vi "Ver 3.0.vi"() -> ()   [LabVIEW 2016]
doc: "This example VI shows how to use thermocouples to take a temperature measurement.\n\nNote:\nFor front panel measurements, make sure the Input switch is in the out position(F)\nFor plug-in card measurements, make sure the Input switch is in the in poisition(R)"
uses:
  Documents/keithley_27xx/Keithley 27XX/Public/Configure/Measurement Specific/Configure FRTD.vi
  Documents/keithley_27xx/Keithley 27XX/Public/Configure/Measurement Specific/Configure Thermocouple.vi
  Documents/keithley_27xx/Keithley 27XX/Public/Configure/Measurement Specific/Configure Thermistor.vi
  Documents/keithley_27xx/Keithley 27XX/Public/Data/Read Multiple Direct.vi
  Documents/keithley_27xx/Keithley 27XX/Keithley 27XX.lvlib
  Documents/keithley_27xx/Keithley 27XX/Public/Close.vi
panel:
  out "Timestamp 12":dbl[](array[numeric])
  out "Timestamp 11":dbl[](array[numeric])
  out "Timestamp 10":dbl[](array[numeric])
  out "Timestamp 9":dbl[](array[numeric])
  out "Timestamp 8":dbl[](array[numeric])
  out "Timestamp 7":dbl[](array[numeric])
  out "Timestamp 6":dbl[](array[numeric])
  out "Timestamp 5":dbl[](array[numeric])
  out "Timestamp 4":dbl[](array[numeric])
  out "Timestamp 3":dbl[](array[numeric])
  out "Timestamp 2":dbl[](array[numeric])
  out "Measurement 12":dbl[](array[numeric])
  out "Measurement 11":dbl[](array[numeric])
  out "Measurement 10":dbl[](array[numeric])
  out "Measurement 9":dbl[](array[numeric])
  out "Measurement 8":dbl[](array[numeric])
  out "Measurement 7":dbl[](array[numeric])
  out "Measurement 6":dbl[](array[numeric])
  out "Measurement 5":dbl[](array[numeric])
  out "Measurement 4":dbl[](array[numeric])
  out "Measurement 3":dbl[](array[numeric])
  out "Measurement 2":dbl[](array[numeric])
  out "Timestamp 1":dbl[](array[numeric])
  out "Measurement 1":dbl[](array[numeric])
  in  "# of Channels":dbl=3.0
  in  "Sample size":dbl=3.0
  in  "Sensor Type":string(combo)="Thermistor"
  in  "Delta1":dbl=1.0
  in  "Beta1":dbl=0.1
  in  "Alpha1":dbl=0.0038
  in  "Serial Configuration":T1={"Baud Rate (9600)"=9600, "Flow Control (1: XON/XOFF)"=1, "Termination Char (0:CR)"=0} {"Termination Char (0:CR)" items=["CR", "LF", "CRLF (Do not use)", "LFCR (Do not use)"]; "Flow Control (1: XON/XOFF)" items=["None", "XON/XOFF", "RTS/CTS (2701 Only)", "XON/XOFF & RTS/CTS (2701 Only)"]; "Baud Rate (9600)" items=["300"=300, "600"=600, "1200"=1200, "2400"=2400, "4800"=4800, "9600"=9600, "19.2k"=19200, "38.4k (2701 Only)"=38400, "57.6k (2701 Only)"=57600, "115.2k (2701 Only)"=115200]}
  in  "VISA resource name":refnum<visa-resource-name>="TCPIP0::192.168.69.200::1394::SOCKET"
  in  "Channels":string="101,102,103"
  in  "Temperature (0: Celsius)":u16(ring) items=["Celsius", "Fahrenheit", "Kelvin"]
  # "*For front panel measurements, make sure the Input switch is in the out position(F)*\n  For plug-in card measurements, make sure the Input switch is in the in position(R)"
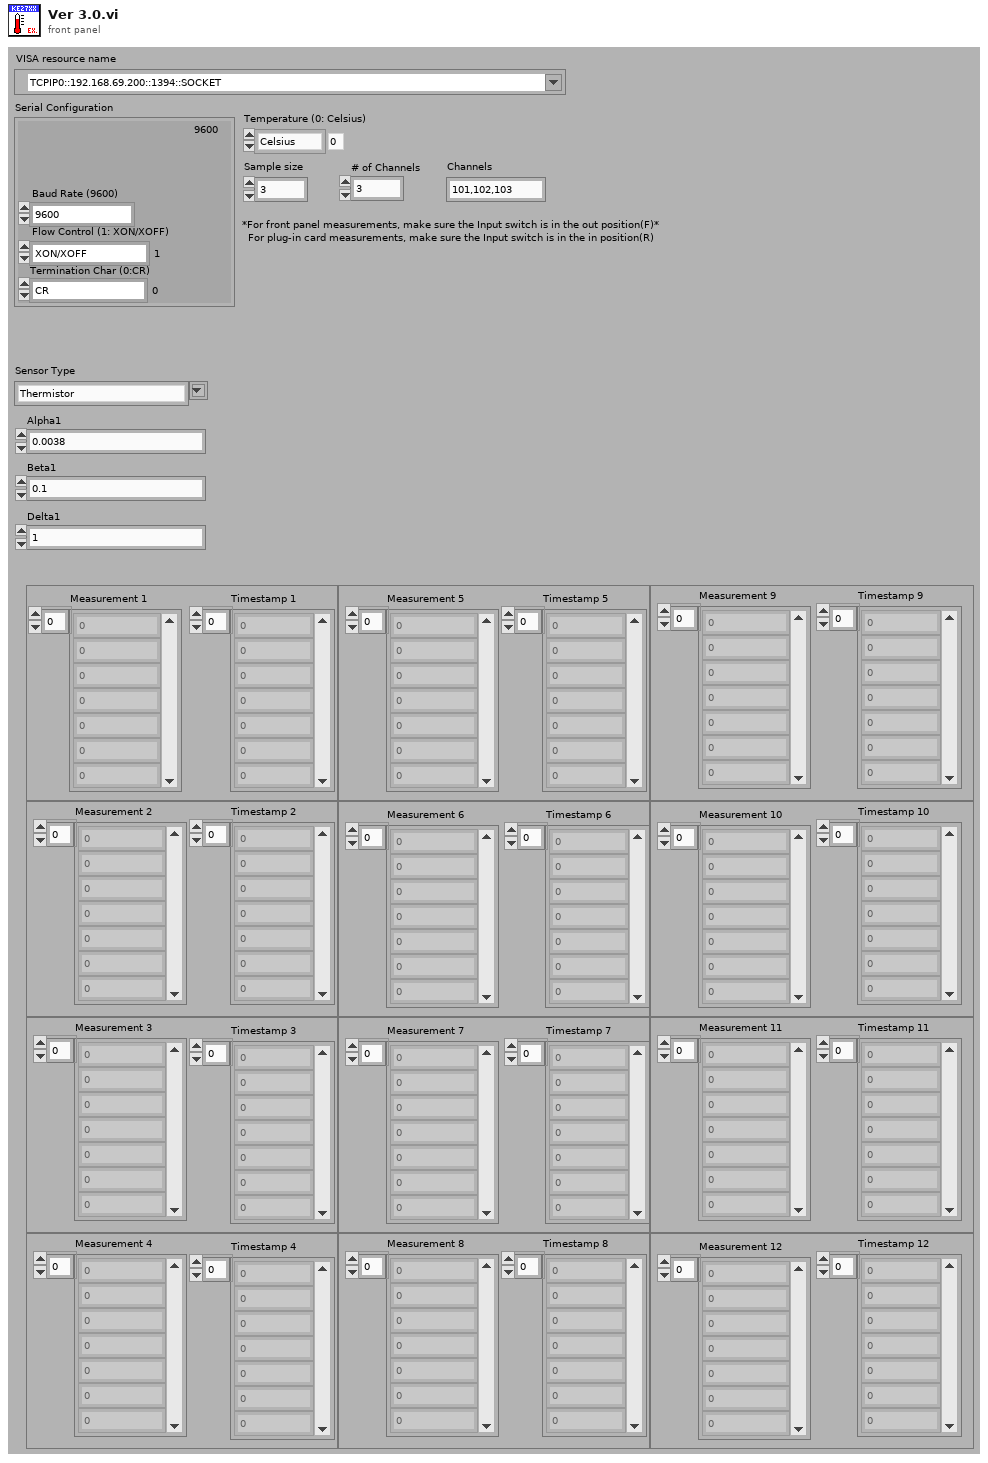
[diagram p1: front panel]
types:
  T1 = cluster{"Baud Rate (9600)":u32, "Flow Control (1: XON/XOFF)":u16, "Termination Char (0:CR)":u16}
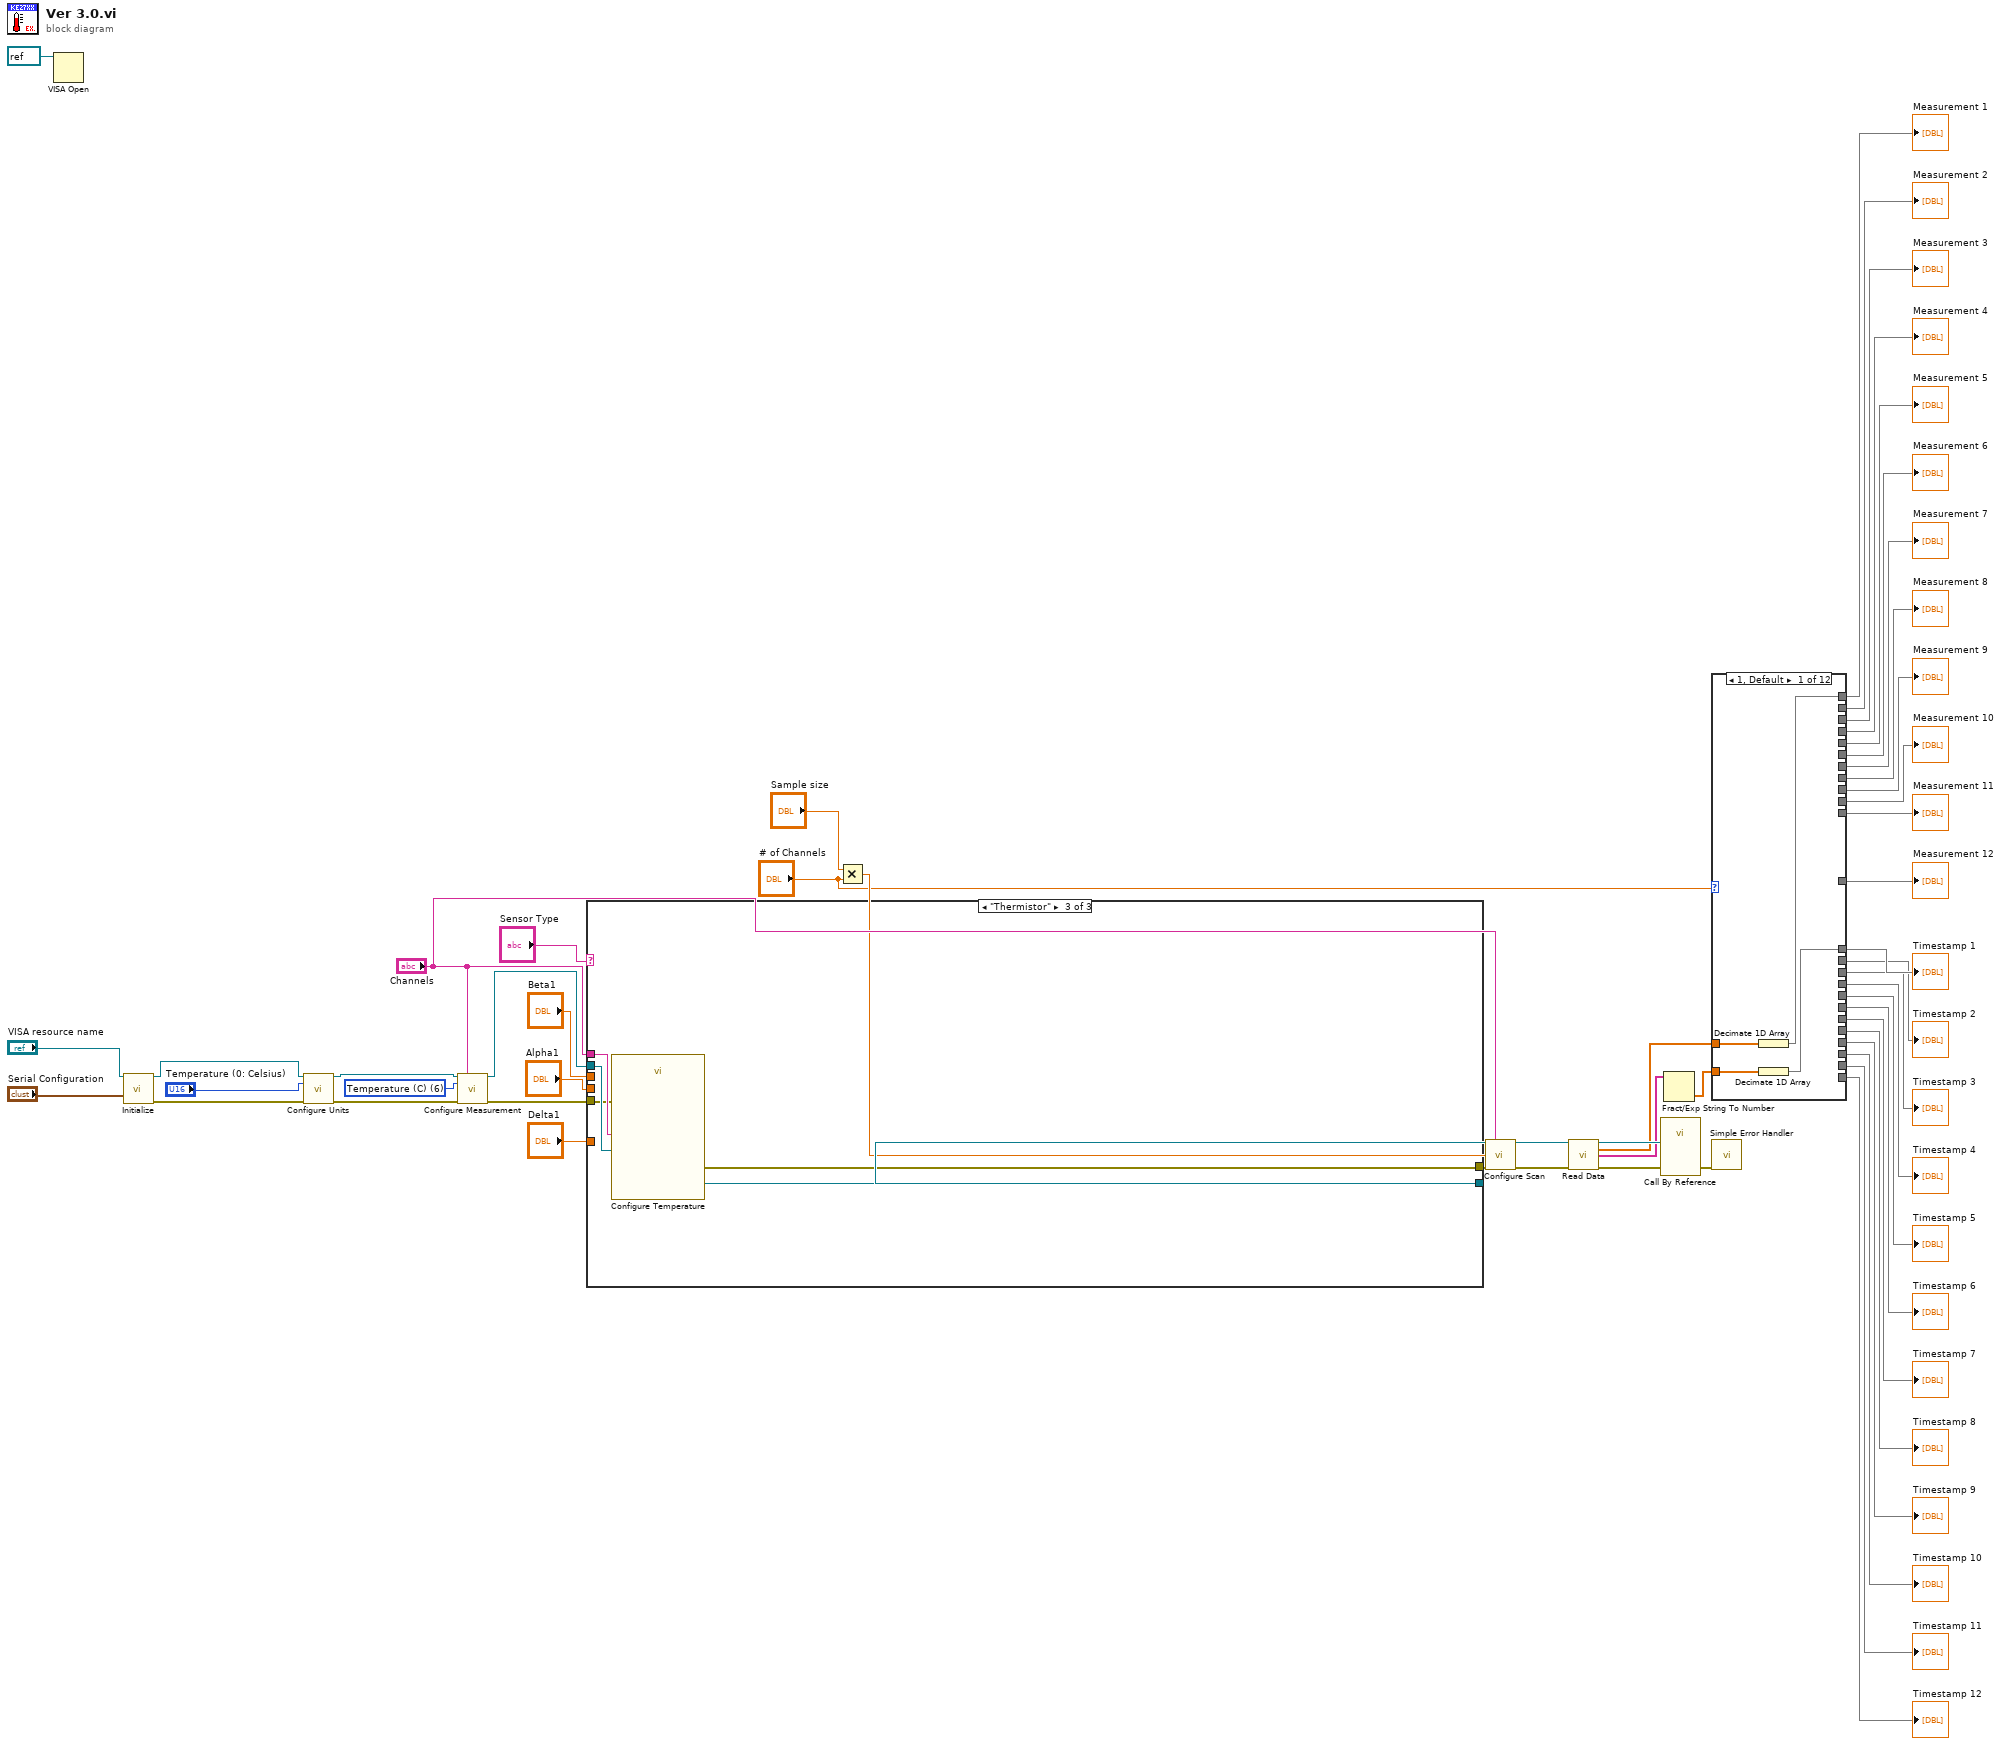
[diagram p0: block diagram]
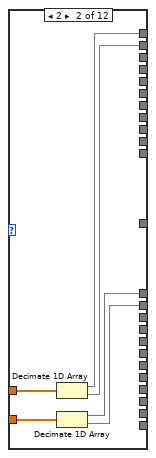
[diagram p2: hidden frame]
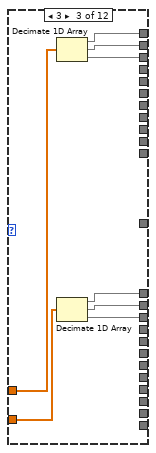
[diagram p3: hidden frame]
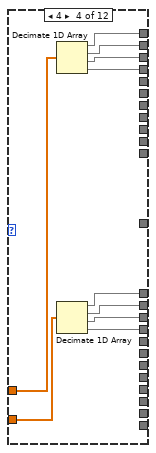
[diagram p4: hidden frame]
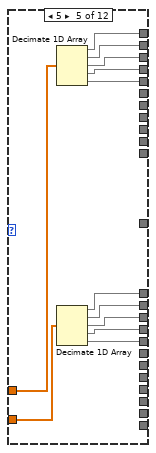
[diagram p5: hidden frame]
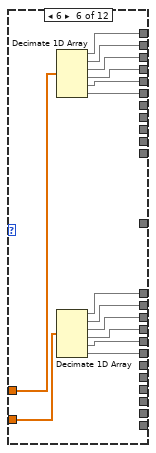
[diagram p6: hidden frame]
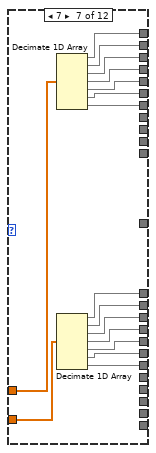
[diagram p7: hidden frame]
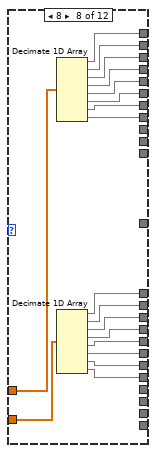
[diagram p8: hidden frame]
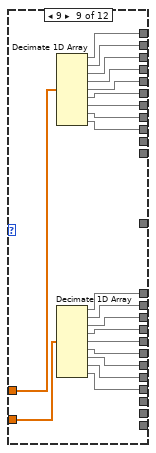
[diagram p9: hidden frame]
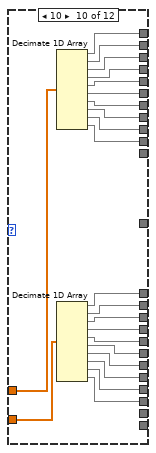
[diagram p10: hidden frame]
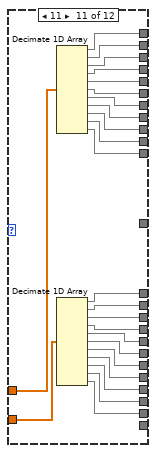
[diagram p11: hidden frame]
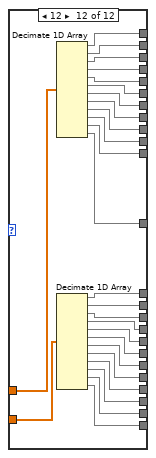
[diagram p12: hidden frame]
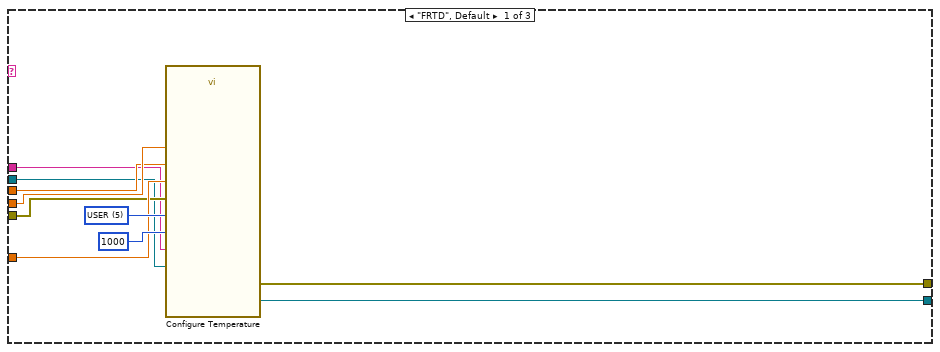
[diagram p13: hidden frame]
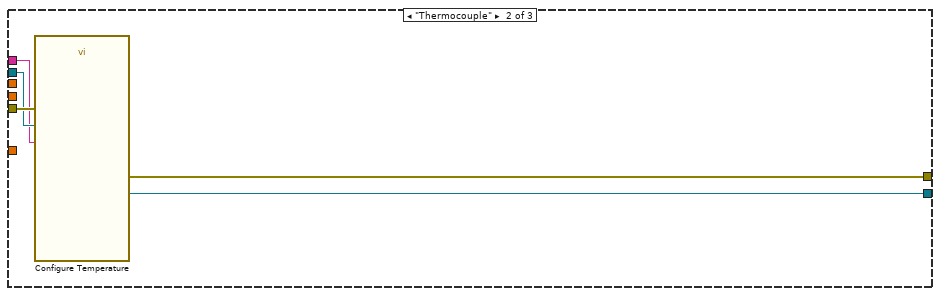
[diagram p14: hidden frame]
diagram:
  w51 = u16 6 items=["DC Voltage", "AC Voltage", "DC Current", "AC Current", "Resistance", "Four-Wire Resistance", "Temperature (C)", "Frequency", "Period", "Continuity"] ("Function (0: DC Voltage)")
  n1 = VISA Open(VISA resource name=refnum<visa-resource-name> refnum) -> ()  [unwired: 4 in, 2 out]
  n2 = call "Initialize.vi"("VISA resource name"="VISA resource name", "Serial Configuration"="Serial Configuration") -> ("VISA resource name out"=w48:refnum<visa-resource-name>, "error out"=w47:errorcluster)  [unwired: 12 in]
  n3 = call "Configure Units.vi"("VISA resource name"=w48, "Temperature (0: Celsius)"="Temperature (0: Celsius)", "error in (no error)"=w47) -> ("VISA resource name out"=w49:refnum<visa-resource-name>, "error out"=w46:errorcluster)  [unwired: 11 in]
  n4 = call "Configure Measurement.vi"("VISA resource name"=w49, "Scan List (Empty)"="Channels", "Function (0: DC Voltage)"=w51, "error in (no error)"=w46) -> ("VISA resource name out"=w38:refnum<visa-resource-name>, "error out"=w39:errorcluster)  [unwired: 10 in]
  n5 = case shown="\"Thermistor\"" "Sensor Type" {
    tunnel: [w62 w67 w73] -> w44
    tunnel: [w63 w68 w72] -> w43
    tunnel: "Delta1" -> [w57 _ _]
    tunnel: "Beta1" -> [w58 _ _]
    tunnel: "Alpha1" -> [w59 _ _]
    tunnel: w39 -> [w56 w66 w69]
    tunnel: w38 -> [w55 w65 w70]
    tunnel: "Channels" -> [w54 w64 w71]
    frame "FRTD", Default {
      w61 = u16 5 items=["PT100", "D100", "F100", "PT3916", "PT385", "USER"] ("FRTD Type (0: PT100)")
      n6 = call-poly "Configure Temperature.vi"("VISA resource name"=w55, "FRTD Type (0: PT100)"=w61, "error in (no error)"=w56, "Scan List (Empty)"=w54, "R Zero (100)"=1000, "Alpha (0.00385)"=w59, "Beta (0.111)"=w58, "Delta (1.507)"=w57) -> ("VISA resource name out"=w63:refnum<visa-resource-name>, "error out"=w62:errorcluster)  [unwired: 10 in]
    }
    frame "Thermocouple" {
      n7 = call-poly "Configure Temperature.vi"("VISA resource name"=w65, "error in (no error)"=w66, "Scan List (Empty)"=w64) -> ("VISA resource name out"=w68:refnum<visa-resource-name>, "error out"=w67:errorcluster)  [unwired: 15 in]
    }
    frame "Thermistor" {
      n8 = call-poly "Configure Temperature.vi"("VISA resource name"=w70, "error in (no error)"=w69, "Scan List (Empty)"=w71) -> ("VISA resource name out"=w72:refnum<visa-resource-name>, "error out"=w73:errorcluster)  [unwired: 15 in]
    }
  }
  n9 = Multiply(x="Sample size", y="# of Channels") -> (x*y=w29:dbl)
  n10 = call "Configure Scan.vi"("VISA resource name"=w43, "Channel List (101:110)"="Channels", "Sample Count (100)"=w29, "error in (no error)"=w44) -> ("VISA resource name out"=w34:refnum<visa-resource-name>, "error out"=w33:errorcluster)  [unwired: 10 in]
  n11 = call-poly "Read Data.vi"("VISA resource name"=w34, "error in (no error)"=w33) -> ("VISA resource name out"=w32:refnum<visa-resource-name>, "Measurement Data"=w31:dbl[], "Time Stamp"=w15:string[], "error out"=w28:errorcluster)  [unwired: 8 in, 2 out]
  n12 = call-by-ref "?"("VISA resource name"=w32, "error in (no error)"=w28) -> ("error out"=w35:errorcluster)  [unwired: 15 in, 2 out]
  n13 = Fract/Exp String To Number(string=w15) -> (number=w26:dbl[])  [unwired: 3 in, 1 out]
  n14 = case shown="1, Default" "# of Channels" {
    tunnel: w26 -> [w77 w82 w90 w100 w112 w126 w142 w160 w180 w202 w226 w252]
    tunnel: w31 -> [w76 w83 w91 w101 w113 w127 w143 w161 w181 w203 w227 w253]
    tunnel: [w75 w81 w89 w99 w111 w125 w141 w159 w179 w201 w225 w251] -> w25
    tunnel: [w74 w80 w86 w96 w108 w122 w138 w156 w176 w198 w222 w248] -> w24
    tunnel: [_ w79 w88 w98 w110 w124 w140 w158 w178 w200 w224 w250] -> w23
    tunnel: [_ w78 w85 w95 w107 w121 w137 w155 w175 w197 w221 w247] -> w22
    tunnel: [_ _ w87 w97 w109 w123 w139 w157 w177 w199 w223 w249] -> w21
    tunnel: [_ _ w84 w94 w106 w120 w136 w154 w174 w196 w220 w246] -> w20
    tunnel: [_ _ _ w93 w105 w119 w135 w153 w173 w195 w219 w245] -> w19
    tunnel: [_ _ _ w92 w104 w118 w134 w152 w172 w194 w218 w244] -> w18
    tunnel: [_ _ _ _ w103 w117 w133 w151 w171 w193 w217 w243] -> w17
    tunnel: [_ _ _ _ w102 w116 w132 w150 w170 w192 w216 w242] -> w16
    tunnel: [_ _ _ _ _ w115 w131 w149 w169 w191 w215 w241] -> w14
    tunnel: [_ _ _ _ _ w114 w130 w148 w168 w190 w214 w240] -> w13
    tunnel: [_ _ _ _ _ _ w129 w147 w167 w189 w213 w239] -> w12
    tunnel: [_ _ _ _ _ _ w128 w146 w166 w188 w212 w238] -> w11
    tunnel: [_ _ _ _ _ _ _ w145 w165 w187 w211 w237] -> w10
    tunnel: [_ _ _ _ _ _ _ w144 w164 w186 w210 w236] -> w9
    tunnel: [_ _ _ _ _ _ _ _ w163 w185 w209 w235] -> w8
    tunnel: [_ _ _ _ _ _ _ _ w162 w184 w208 w234] -> w7
    tunnel: [_ _ _ _ _ _ _ _ _ w183 w207 w233] -> w6
    tunnel: [_ _ _ _ _ _ _ _ _ w182 w206 w232] -> w5
    tunnel: [_ _ _ _ _ _ _ _ _ _ w205 w231] -> w4
    tunnel: [_ _ _ _ _ _ _ _ _ _ w204 w230] -> w3
    tunnel: [_ _ _ _ _ _ _ _ _ _ _ w229] -> w2
    tunnel: [_ _ _ _ _ _ _ _ _ _ _ w228] -> w1
    frame 1, Default {
      n15 = Decimate 1D Array(w76) -> (w75:dbl[])
      n16 = Decimate 1D Array(w77) -> (w74:dbl[])
    }
    frame 2 {
      n17 = Decimate 1D Array(w83) -> (w81:dbl[], w79:dbl[])
      n18 = Decimate 1D Array(w82) -> (w80:dbl[], w78:dbl[])
    }
    frame 3 {
      n19 = Decimate 1D Array(w91) -> (w89:dbl[], w88:dbl[], w87:dbl[])
      n20 = Decimate 1D Array(w90) -> (w86:dbl[], w85:dbl[], w84:dbl[])
    }
    frame 4 {
      n21 = Decimate 1D Array(w101) -> (w99:dbl[], w98:dbl[], w97:dbl[], w93:dbl[])
      n22 = Decimate 1D Array(w100) -> (w96:dbl[], w95:dbl[], w94:dbl[], w92:dbl[])
    }
    frame 5 {
      n23 = Decimate 1D Array(w113) -> (w111:dbl[], w110:dbl[], w109:dbl[], w105:dbl[], w103:dbl[])
      n24 = Decimate 1D Array(w112) -> (w108:dbl[], w107:dbl[], w106:dbl[], w104:dbl[], w102:dbl[])
    }
    frame 6 {
      n25 = Decimate 1D Array(w127) -> (w125:dbl[], w124:dbl[], w123:dbl[], w119:dbl[], w117:dbl[], w115:dbl[])
      n26 = Decimate 1D Array(w126) -> (w122:dbl[], w121:dbl[], w120:dbl[], w118:dbl[], w116:dbl[], w114:dbl[])
    }
    frame 7 {
      n27 = Decimate 1D Array(w143) -> (w141:dbl[], w140:dbl[], w139:dbl[], w135:dbl[], w133:dbl[], w131:dbl[], w129:dbl[])
      n28 = Decimate 1D Array(w142) -> (w138:dbl[], w137:dbl[], w136:dbl[], w134:dbl[], w132:dbl[], w130:dbl[], w128:dbl[])
    }
    frame 8 {
      n29 = Decimate 1D Array(w161) -> (w159:dbl[], w158:dbl[], w157:dbl[], w153:dbl[], w151:dbl[], w149:dbl[], w147:dbl[], w145:dbl[])
      n30 = Decimate 1D Array(w160) -> (w156:dbl[], w155:dbl[], w154:dbl[], w152:dbl[], w150:dbl[], w148:dbl[], w146:dbl[], w144:dbl[])
    }
    frame 9 {
      n31 = Decimate 1D Array(w181) -> (w179:dbl[], w178:dbl[], w177:dbl[], w173:dbl[], w171:dbl[], w169:dbl[], w167:dbl[], w165:dbl[], w163:dbl[])
      n32 = Decimate 1D Array(w180) -> (w176:dbl[], w175:dbl[], w174:dbl[], w172:dbl[], w170:dbl[], w168:dbl[], w166:dbl[], w164:dbl[], w162:dbl[])
    }
    frame 10 {
      n33 = Decimate 1D Array(w203) -> (w201:dbl[], w200:dbl[], w199:dbl[], w195:dbl[], w193:dbl[], w191:dbl[], w189:dbl[], w187:dbl[], w185:dbl[], w183:dbl[])
      n34 = Decimate 1D Array(w202) -> (w198:dbl[], w197:dbl[], w196:dbl[], w194:dbl[], w192:dbl[], w190:dbl[], w188:dbl[], w186:dbl[], w184:dbl[], w182:dbl[])
    }
    frame 11 {
      n35 = Decimate 1D Array(w227) -> (w225:dbl[], w224:dbl[], w223:dbl[], w219:dbl[], w217:dbl[], w215:dbl[], w213:dbl[], w211:dbl[], w209:dbl[], w207:dbl[], w205:dbl[])
      n36 = Decimate 1D Array(w226) -> (w222:dbl[], w221:dbl[], w220:dbl[], w218:dbl[], w216:dbl[], w214:dbl[], w212:dbl[], w210:dbl[], w208:dbl[], w206:dbl[], w204:dbl[])
    }
    frame 12 {
      n37 = Decimate 1D Array(w253) -> (w251:dbl[], w250:dbl[], w249:dbl[], w245:dbl[], w243:dbl[], w241:dbl[], w239:dbl[], w237:dbl[], w235:dbl[], w233:dbl[], w231:dbl[], w229:dbl[])
      n38 = Decimate 1D Array(w252) -> (w248:dbl[], w247:dbl[], w246:dbl[], w244:dbl[], w242:dbl[], w240:dbl[], w238:dbl[], w236:dbl[], w234:dbl[], w232:dbl[], w230:dbl[], w228:dbl[])
    }
  }
  "Measurement 1" <- w25
  "Timestamp 1" <- w24
  "Measurement 2" <- w23
  "Measurement 3" <- w21
  "Measurement 4" <- w19
  "Measurement 5" <- w17
  "Measurement 6" <- w14
  "Measurement 7" <- w12
  "Measurement 8" <- w10
  "Measurement 9" <- w8
  "Measurement 10" <- w6
  "Measurement 11" <- w4
  "Measurement 12" <- w2
  "Timestamp 2" <- w22
  "Timestamp 3" <- w20
  "Timestamp 4" <- w18
  "Timestamp 5" <- w16
  "Timestamp 6" <- w13
  "Timestamp 7" <- w11
  "Timestamp 8" <- w9
  "Timestamp 9" <- w7
  "Timestamp 10" <- w5
  "Timestamp 11" <- w3
  "Timestamp 12" <- w1
  n39 = call <vilib>:"Simple Error Handler.vi"("error in (no error)"=w35) -> ()  [unwired: 4 in, 5 out]
